vi "queueImages.vi"(0 "buffer number":u32, 1 "buffer iteration":i32, 2 "buffer index":i32, 3 "rectangle":i32[](array[numeric])) -> ()   [LabVIEW 2012]
uses:
  GlobalBaslerCamera.vi
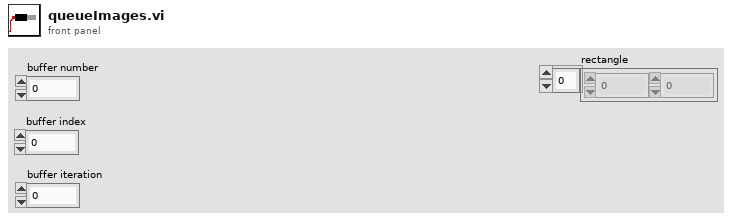
[diagram p1: front panel]
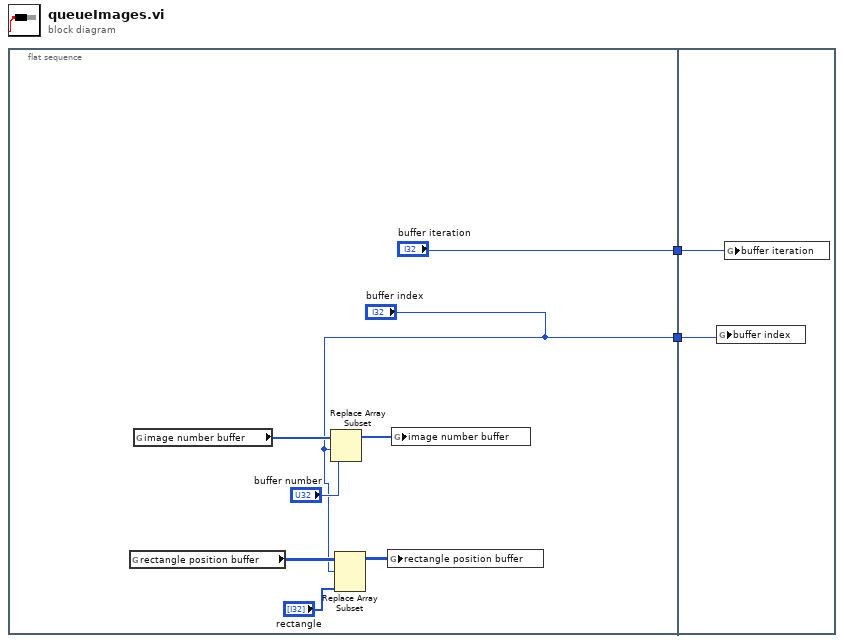
[diagram p0: block diagram]
diagram:
  n1 = flat-sequence {
    tunnel: ["buffer index"] -> w2
    tunnel: ["buffer iteration"] -> w1
    tunnel: w2 -> [w12]
    tunnel: w1 -> [w11]
    frame #0 {
      n2 = global read "GlobalBaslerCamera.vi" "rectangle position buffer"() -> (w7:u16[][])
      n3 = global read "GlobalBaslerCamera.vi" "image number buffer"() -> (w10:u16[])
      n4 = Replace Array Subset(array=w10, new element="buffer number", index="buffer index") -> (w8:u16[])
      n5 = Replace Array Subset(array=w7, new element="rectangle", index (row)="buffer index") -> (w6:u16[][])  [unwired: 1 in]
      n6 = global write "GlobalBaslerCamera.vi" "rectangle position buffer"(w6) -> ()
      n7 = global write "GlobalBaslerCamera.vi" "image number buffer"(w8) -> ()
    }
    frame #1 {
      n8 = global write "GlobalBaslerCamera.vi" "buffer index"(w12) -> ()
      n9 = global write "GlobalBaslerCamera.vi" "buffer iteration"(w11) -> ()
    }
  }
